vi "Ref_Num_OverrideSpec.vi"(8 "error in":errorcluster, 10 "Specific Frequency":refnum<vi>, 11 "Set LCR Frequency":refnum<vi>) -> (0 "error out":errorcluster)   [LabVIEW 2020]
uses:
  Global 1.vi
panel:
  # "Manual Override :\nSet Specific Frequency\nafter choosing TSL"
  # "Get 4275A Keystate"
  # "This is for Resetting, from \nGlobal Variable"
  # "[] [AN] [BN] [CN] [DN] [FNN]"
  # "0 - NULL  -   \n1-  10kHz             - F11\n2-  20(30) kHz     - F12 \n3-  40(50) kHz     - F13\n4-  100 kHz          - F14\n5-  200(300) kHz - F15\n6-  400(500) kHz - F16\n7-  1 MHz            - F17\n8-  2(3) MHz       - F18\n9-  4(5) MHz       - F19\n10- 10 MHz         - F20\n11- *1                   - F21\n12- *2                   - F22"
  # "Frequency Step\n10 kHz - F11                     1 MHz - F17\n20(30) kHz - F12              2(3) MHz - F18\n40(50) kHz - F13              4(5) MHz - F19\n100 kHz - F14                   10 MHz - F20\n200(300) kHz - F15           *1 - F21\n400(500) kHz - F16           *2 - F22"
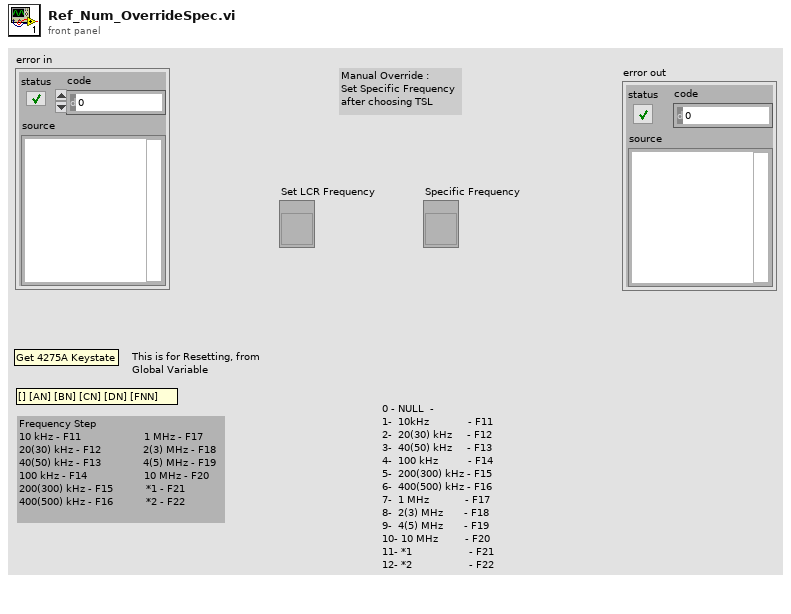
[diagram p1: front panel]
types:
  T1 = enum16{"NULL", "10kHz", "20(30)kHz", "40(50)kHz", "100kHz", "200(300)kHz", "400(500)kHz", "1MHz", "2(3)MHz", "4(5)MHz", "10MHz", "*1", "*2"}
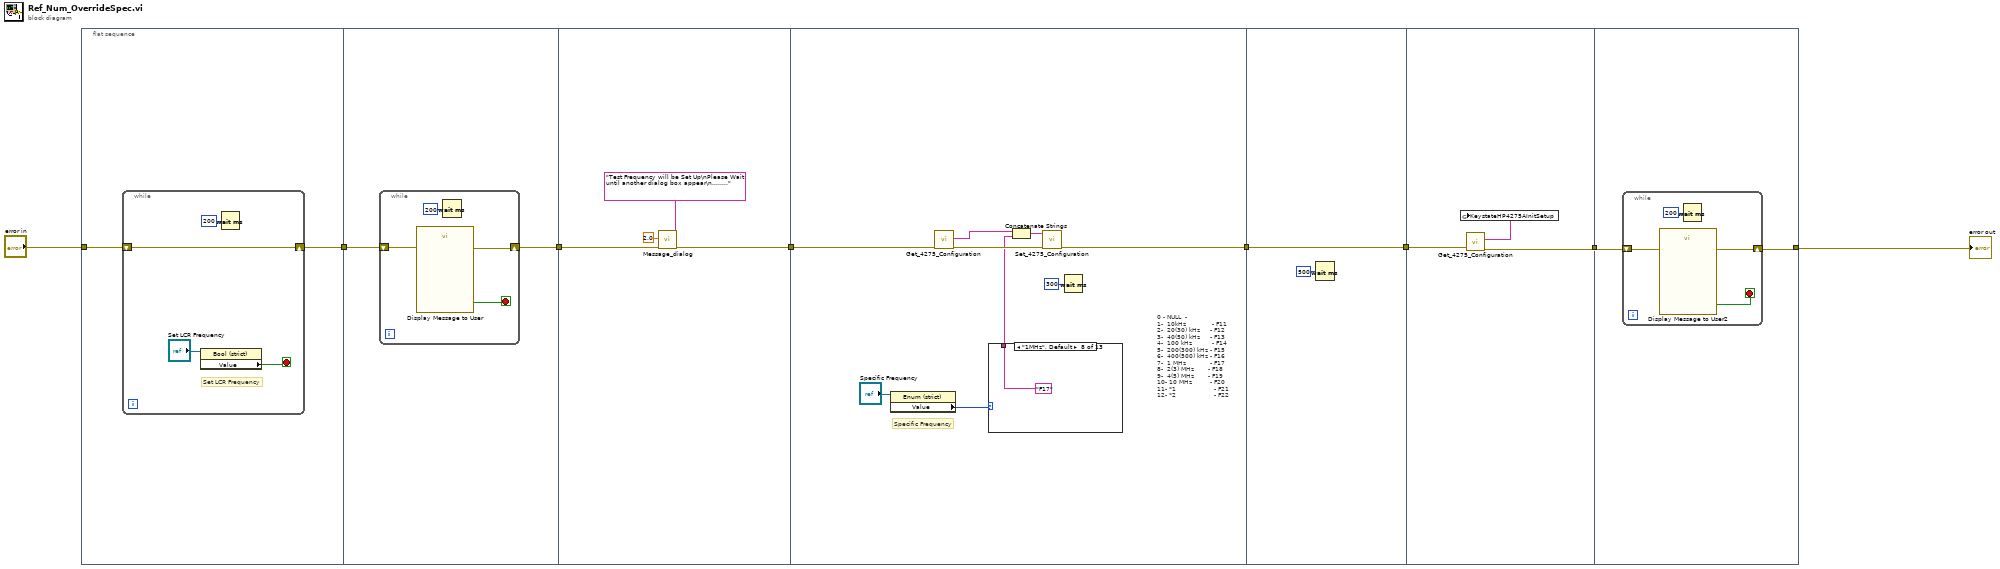
[diagram p0: block diagram]
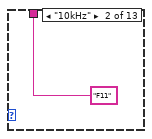
[diagram p3: hidden frame]
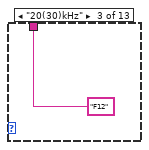
[diagram p4: hidden frame]
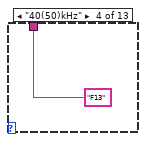
[diagram p5: hidden frame]
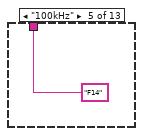
[diagram p6: hidden frame]
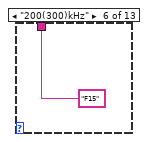
[diagram p7: hidden frame]
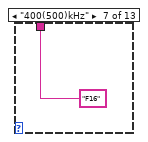
[diagram p8: hidden frame]
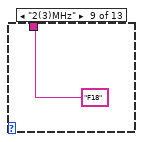
[diagram p9: hidden frame]
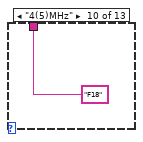
[diagram p10: hidden frame]
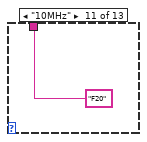
[diagram p11: hidden frame]
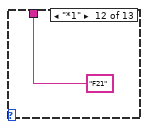
[diagram p12: hidden frame]
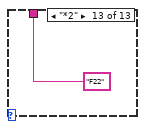
[diagram p13: hidden frame]
diagram:
  n1 = flat-sequence {
    tunnel: "error in" -> [w10]
    tunnel: [w9] -> w8
    tunnel: w8 -> [w16]
    tunnel: [w15] -> w7
    tunnel: w7 -> [w22]
    tunnel: [w21] -> w6
    tunnel: w6 -> [w30]
    tunnel: [w28] -> w5
    tunnel: w5 -> [w47]
    tunnel: [w47] -> w4
    tunnel: w4 -> [w49]
    tunnel: [w48] -> w3
    tunnel: [w51] -> w1
    tunnel: w3 -> [w52]
    frame #0 {
      n2 = while {
        shift-right: [w14] -> w9
        shift-left: w10 -> [w14]
        stop <- w12 stop-if-true
        # "Set LCR Frequency"
        n3 = property class="Bool (strict)"(reference="Set LCR Frequency") -> ("Value"=w12:bool)  [unwired: 1 in, 2 out]
        n4 = Wait (ms)(milliseconds to wait=u32 200) -> ()  [unwired: 1 out]
      }
    }
    frame #1 {
      n5 = while {
        shift-right: [w18] -> w15
        shift-left: w16 -> [w19]
        stop <- w20 stop-if-true
        n6 = call "Display Message to User"("error in (no error)"=w19) -> ("error out"=w18:errorcluster, "YES"=w20:bool)  [unwired: 9 in]
        n7 = Wait (ms)(milliseconds to wait=u32 200) -> ()  [unwired: 1 out]
      }
    }
    frame #2 {
      n8 = call "Message_dialog.vi"("error in (no error)"=w22, "set delay"=2.0, "String"="Test Frequency will be Set Up\nPlease Wait until another dialog box appear\n........") -> ("error out"=w21:errorcluster)  [unwired: 8 in]
    }
    frame #3 {
      # "Specific Frequency"
      # "0 - NULL  -   \n1-  10kHz             - F11\n2-  20(30) kHz     - F12 \n3-  40(50) kHz     - F13\n4-  100 kHz          - F14\n5-  200(300) kHz - F15\n6-  400(500) kHz - F16\n7-  1 MHz            - F17\n8-  2(3) MHz       - F18\n9-  4(5) MHz       - F19\n10- 10 MHz         - F20\n11- *1                   - F21\n12- *2                   - F22"
      n9 = property class="Enum (strict)"(reference="Specific Frequency") -> ("Value"=w26:T1)  [unwired: 1 in, 2 out]
      n10 = call "Get_4275_Configuration.vi"("error in"=w30) -> ("error out"=w31:errorcluster, "Keystate"=w33:string)  [unwired: 9 in]
      n11 = case shown="\"1MHz\", Default" w26 {
        tunnel: [_ "F11" ("string") "F12" ("string") "F13" ("string") "F14" ("string") "F15" ("string") "F16" ("string") "F17" ("string") "F18" ("string") "F18" ("string") "F20" ("string") "F21" ("string") "F22" ("string")] -> w29
        frame "NULL" {
        }
        frame "10kHz" {
        }
        frame "20(30)kHz" {
        }
        frame "40(50)kHz" {
        }
        frame "100kHz" {
        }
        frame "200(300)kHz" {
        }
        frame "400(500)kHz" {
        }
        frame "1MHz", Default {
        }
        frame "2(3)MHz" {
        }
        frame "4(5)MHz" {
        }
        frame "10MHz" {
        }
        frame "*1" {
        }
        frame "*2" {
        }
      }
      n12 = Concatenate Strings(w33, w29) -> (w32:string)
      n13 = call "Set_4275_Configuration.vi"("error in"=w31, "Keystate"=w32) -> ("error out"=w28:errorcluster)  [unwired: 9 in]
      n14 = Wait (ms)(milliseconds to wait=u32 300) -> ()  [unwired: 1 out]
    }
    frame #4 {
      n15 = Wait (ms)(milliseconds to wait=u32 500) -> ()  [unwired: 1 out]
    }
    frame #5 {
      n16 = call "Get_4275_Configuration.vi"("error in"=w49) -> ("error out"=w48:errorcluster, "Keystate"=w50:string)  [unwired: 9 in]
      n17 = global write "Global 1.vi" "KeystateHP4275AInitSetup"(w50) -> ()
    }
    frame #6 {
      n18 = while {
        shift-right: [w54] -> w51
        shift-left: w52 -> [w55]
        stop <- w56 stop-if-true
        n19 = call "Display Message to User2"("error in (no error)"=w55) -> ("error out"=w54:errorcluster, "OK"=w56:bool)  [unwired: 9 in]
        n20 = Wait (ms)(milliseconds to wait=u32 200) -> ()  [unwired: 1 out]
      }
    }
  }
  "error out" <- w1
